vi "MCB2400 AI Specify Node.vi"(10 "Node Attributes":T2, 11 "Attributes":T1 {"Programmable Pin Connections" items=["AI0 uses pin P0.23. You cannot use AI0 and pin P0.23 in the same project.", "AI1 uses pin P0.24. You cannot use AI1 and pin P0.24 in the same project. ", "AI2 uses pin P0.25. You cannot use AI2 and pin P0.25 in the same project.", "AI3 uses pin P0.26 (also used by AOUT). You cannot use AI3 and pin P0.26 (or AOUT) in the same project.", "AI4 uses pin P1.30. You cannot use AI4 and pin P1.30 in the same project.", "AI5 uses pin P1.31. You cannot use AI5 and pin P1.31 in the same project.", "AI6 uses pin P0.12. You cannot use AI6 and pin P0.12 in the same project.", "AI7 uses pin P0.13. You cannot use AI7 and pin P0.13 in the same project."]}) -> (3 "type out":T3)   [LabVIEW 2011]
doc: "This VI is a \"Specify Node\" vi. It is used to pick which I/O Implementation VI to use when more than one is specified for an I/O resource. This VI looks at the Node Attributes and selects the type of the I/O based on whether the user selects array or scalar data and whether they select scaled or raw binary. The output is a variant that indicates the type returned by the I/O and it must match the type of one of the I/O Implementation VIs."
uses:
  <vilib>/eio/EIO_TypeDescriptor.ctl
  <vilib>/Embedded/ARM/MCB2400/MCB2400_AI_NodeAttr.ctl
  <vilib>/Embedded/ARM/MCB2400/MCB2400_AI_PrjAttr.ctl
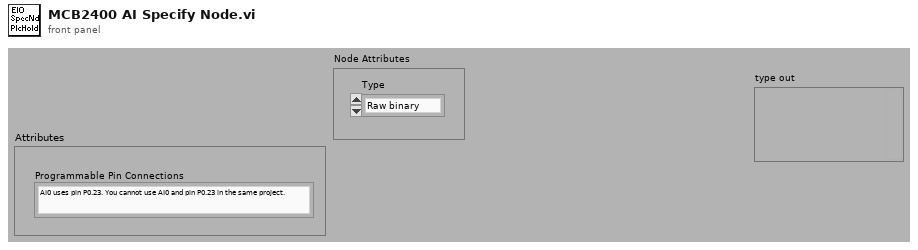
[diagram p1: front panel]
types:
  T1 = typedef "MCB2400_AI_PrjAttr.ctl" = cluster{"Programmable Pin Connections":u16}
  T2 = typedef "MCB2400_AI_NodeAttr.ctl" = cluster{"Type":enum16{"Raw binary", "Scaled voltage"}}
  T3 = typedef "EIO_TypeDescriptor.ctl" = variant
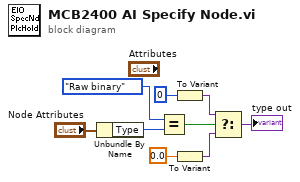
[diagram p0: block diagram]
diagram:
  n1 = Unbundle By Name("Node Attributes") -> ("Type"=w5:enum16{"Raw binary", "Scaled voltage"})
  n2 = Equal?(x=enum16{"Raw binary", "Scaled voltage"}."Raw binary" ("Type"), y=w5) -> (x = y?=w4:bool)
  n3 = To Variant(anything=u16 0) -> (Variant=w7:variant)
  n4 = To Variant(anything=0.0) -> (Variant=w8:variant)
  n5 = Select(t=w7, s=w4, f=w8) -> (s? t:f=→"type out":variant)
